vi "PKG_IMC_SetCompenInfo.vi"(1 "axis":i32, 4 "dist":i32, 5 "dec":dbl, 6 "acc":dbl, 7 "tgvel":dbl, 9 "endvel":dbl, 10 "startvel":dbl, 11 "handle":u32) -> (2 "function return":i32, 3 "handle out":u32)   [LabVIEW 2011, in "IMC_Pkg4xxx.lvlib"]
doc: "PKG_IMC_SetCompenInfo(IMC_HANDLE handle, double startvel, double endvel, double tgvel, double acc, double dec, long dist, int axis);"
uses:
  IMC_Pkg4xxx.lvlib
  IMC_Pkg4xxx.dll
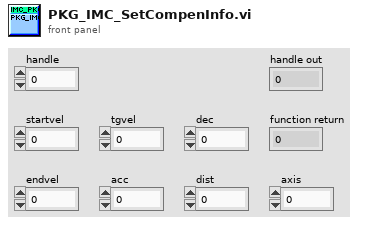
[diagram p1: front panel]
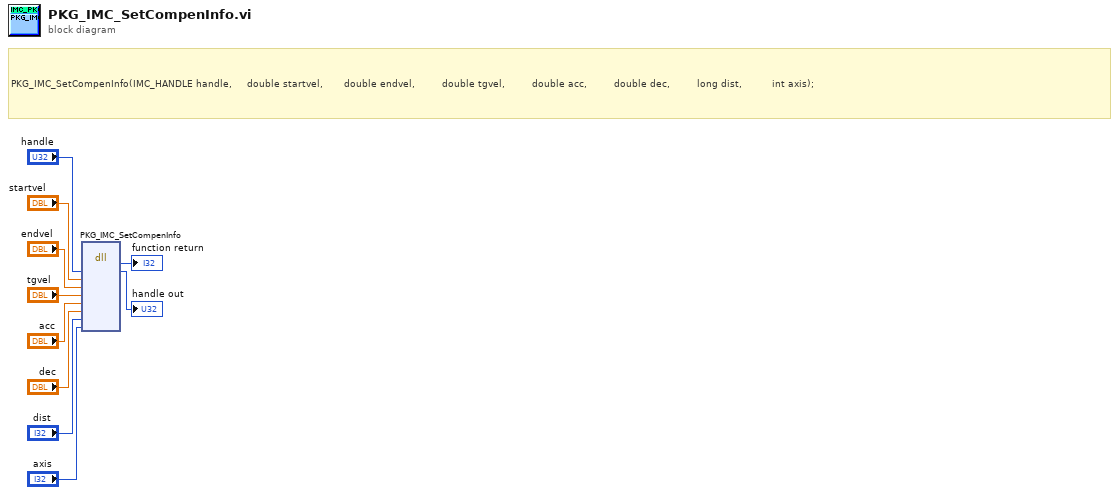
[diagram p0: block diagram]
diagram:
  # "PKG_IMC_SetCompenInfo(IMC_HANDLE handle,\t\t\t\t\tdouble startvel,\t\t\t\t\t\t\tdouble endvel, \t\t\t\t\t\t\t\tdouble tgvel, \t\t\t\t\t\t\t\tdouble acc, \t\t\t\t\t\t\t\tdouble dec, \t\t\t\t\t\t\t\tlong dist, \t\t\t\t\t\t\t\t\tint axis);"
  n1 = dll-call lib="PTH1mabs F光盘刻录\niMC MotionIMCNet_V4.0IMCAppincLabviewIMC_PKG4xxxIMC_PKG4xxx\nIMC_Pkg4xxx.*" fn="PKG_IMC_SetCompenInfo"("handle"="handle", "startvel"="startvel", "endvel"="endvel", "tgvel"="tgvel", "acc"="acc", "dec"="dec", "dist"="dist", "axis"="axis") -> (→"function return":i32, "handle"=→"handle out":u32)  [unwired: 10 in, 2 out]
